vi "replace cursor - plot ref - V2.vi"(0 "Plot ref in":refnum<vi>, 1 "new X":dbl=nan, 3 "new  Y":dbl=nan, 5 "cursor index":i32, 6 "cursor action":T1=enum."write", 7 "label":enum16{"hide", "show x", "show y", "show (x,y)"}(ring), 9 "x-label":string, 11 "y-label":string, 12 "Color Box":u32(colorbox)=327424, 13 "cursor state":T2(ring)=enum."boring") -> (14 "Plot ref out":refnum<vi>, 15 "read X":dbl, 18 "read Y":dbl)   [LabVIEW 2015]
uses:
  cursor action.ctl
panel:
  in  "action":enum16{"", "read", "write"}(ring)=enum."write"
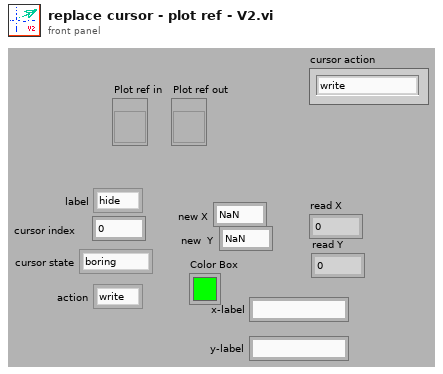
[diagram p1: front panel]
types:
  T1 = typedef "cursor action.ctl" = enum16{"range", "read", "write", "check", "zoom out", "smart zoom out"}
  T2 = enum16{"normal", "alert", "fuzzy", "interesting", "boring", "colored"}
  T3 = typedef "LVCursorListTypeDef.ctl" = cluster{"Name":string, "Color":u32, "Style":u8, "Point Style":u8, "Name Visible":bool, "Allow Drag":bool, "Cursor Mode":u32, "Plot":i32, "Index":i32, "Position":cluster{"X":dbl, "Y":dbl}, "X Scale":u32, "Y Scale":u32, "Watch Plots":i32[], "Watch All Plots":bool, "Plot Area":i32, "Label Offset":cluster{"X":dbl, "Y":dbl}}[]
  T4 = cluster{"Name":string, "Color":u32, "Style":u8, "Point Style":u8, "Name Visible":bool, "Allow Drag":bool, "Cursor Mode":u32, "Plot":i32, "Index":i32, "Position":cluster{"X":dbl, "Y":dbl}, "X Scale":u32, "Y Scale":u32, "Watch Plots":i32[], "Watch All Plots":bool, "Plot Area":i32, "Label Offset":cluster{"X":dbl, "Y":dbl}}
  T5 = typedef "LVRangeTypeDef.ctl" = cluster{"Minimum":dbl, "Maximum":dbl, "Increment":dbl, "Minor Increment":dbl, "Start":dbl}
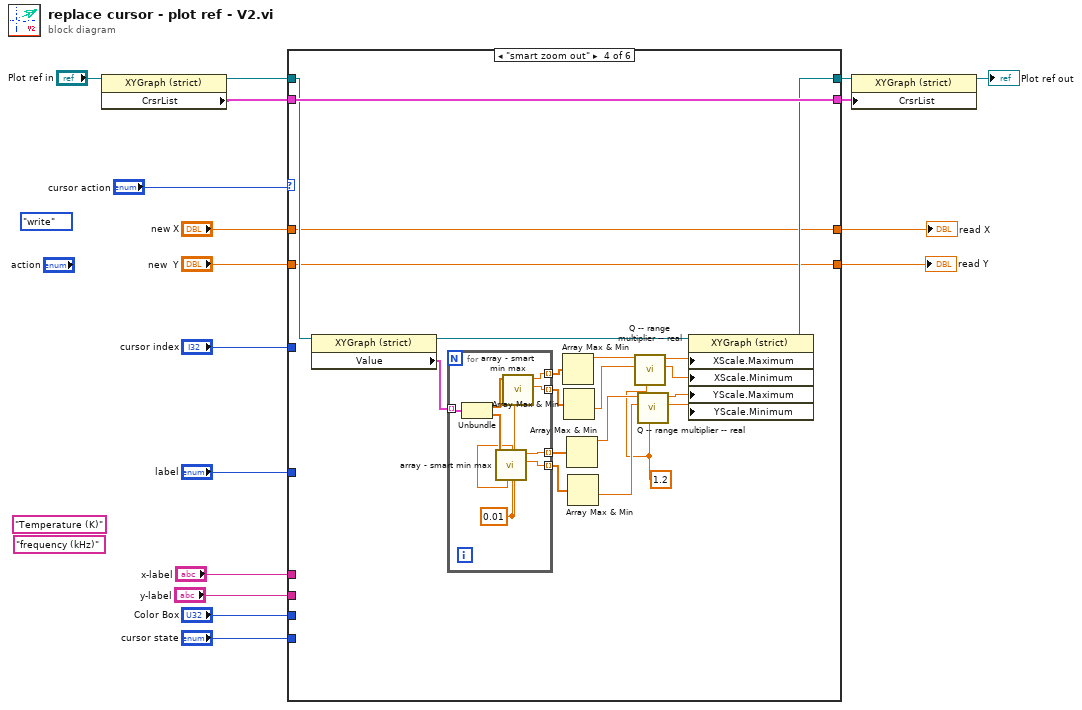
[diagram p0: block diagram]
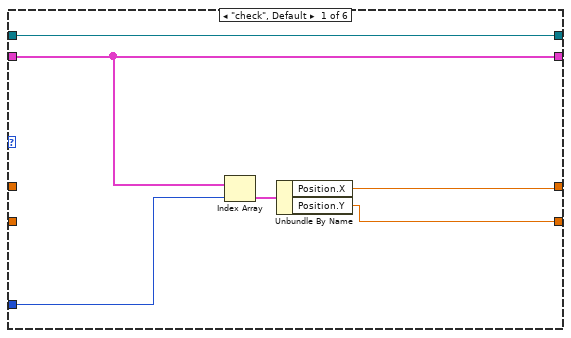
[diagram p2: hidden frame]
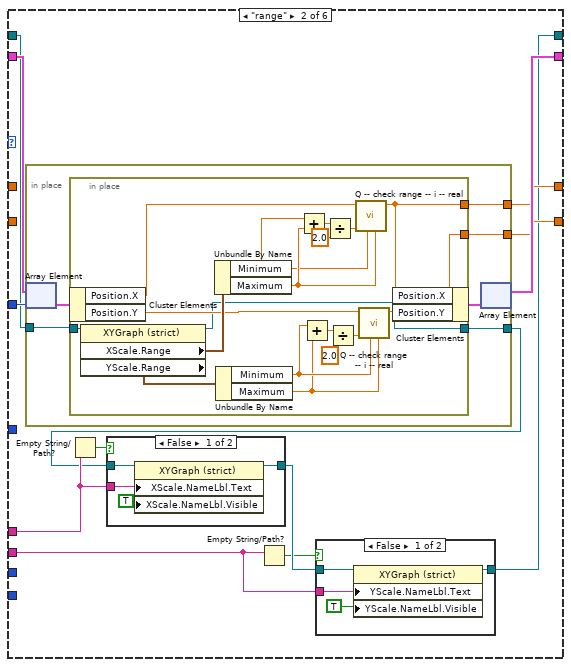
[diagram p3: hidden frame]
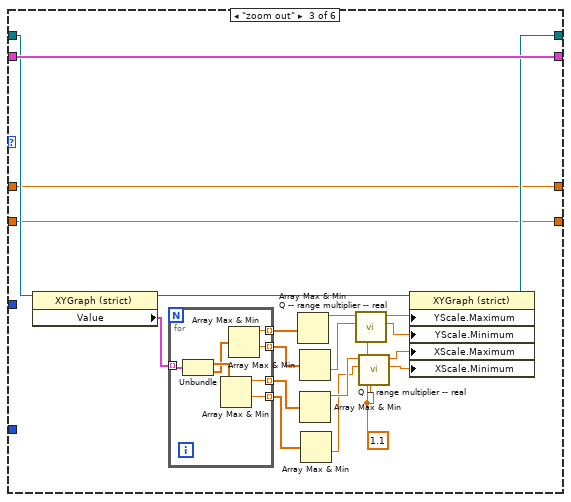
[diagram p6: hidden frame]
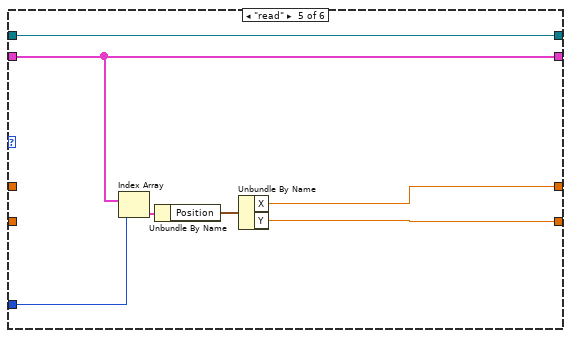
[diagram p7: hidden frame]
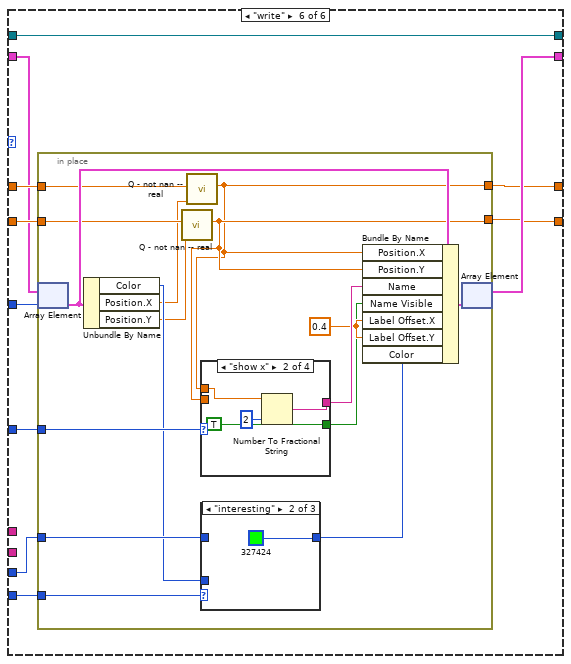
[diagram p8: hidden frame]
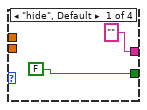
[diagram p11: hidden frame]
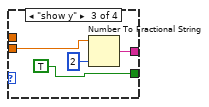
[diagram p12: hidden frame]
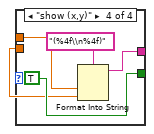
[diagram p13: hidden frame]
diagram:
  (unwired) "frequency (kHz)"
  (unwired) "Temperature (K)"
  (unwired) cursor_action."write" ("cursor action")
  n1 = property on="Property Node" class="XYGraph (strict)"(reference="Plot ref in") -> (reference out=w3:refnum<vi>, "CrsrList"=w12:T3)  [unwired: 1 in, 1 out]
  n2 = case shown="\"smart zoom out\"" "cursor action" {
    tunnel: "cursor index" -> [w21 w34 _ _ w131 w139]
    tunnel: w12 -> [w22 w36 w90 w117 w129 w141]
    tunnel: [w22 w35 w90 w117 w129 w140] -> w11
    tunnel: "new  Y" -> [_ _ w85 w112 _ w142]
    tunnel: "new X" -> [_ _ w86 w113 _ w143]
    tunnel: [w19 w33 w86 w113 w128 w138] -> w14
    tunnel: [w18 w32 w85 w112 w127 w137] -> w13
    tunnel: "label" -> [_ _ _ _ _ w136]
    tunnel: "Color Box" -> [_ _ _ _ _ w135]
    tunnel: "cursor state" -> [_ _ _ _ _ w134]
    tunnel: [w23 w24 w87 w114 w126 w133] -> w4
    tunnel: w3 -> [w23 w31 w89 w116 w126 w133]
    tunnel: "x-label" -> [_ w29 _ _ _ _]
    tunnel: "y-label" -> [_ w26 _ _ _ _]
    frame "check", Default {
      n3 = Index Array(array=w22, index=w21) -> (element=w20:T4)
      n4 = Unbundle By Name(w20) -> ("Position.X"=w19:dbl, "Position.Y"=w18:dbl)
    }
    frame "range" {
      n5 = in-place {
        in-place-border: w31 -> [w50]
        in-place-border: [w49] -> w33
        in-place-border: [w48] -> w32
        in-place-border: [w47] -> w25
        n6 = in-place-array #1(w36, w34) -> (w52:T4)
        n7 = in-place {
          in-place-border: w50 -> [w58]
          in-place-border: [w55] -> w49
          in-place-border: [w54] -> w48
          in-place-border: [w53] -> w47
          n8 = in-place-cluster #2(w52) -> ("Position.X"=w57:dbl, "Position.Y"=w56:dbl)
          n9 = property on="Property Node" class="XYGraph (strict)"(reference=w58) -> (reference out=w53:refnum<vi>, "XScale.Range"=w59:T5, "YScale.Range"=w60:T5)  [unwired: 1 in, 1 out]
          n10 = Unbundle By Name(w59) -> ("Minimum"=w61:dbl, "Maximum"=w62:dbl)
          n11 = Unbundle By Name(w60) -> ("Minimum"=w70:dbl, "Maximum"=w69:dbl)
          n12 = Add(x=w61, y=w62) -> (x+y=w63:dbl)
          n13 = Add(x=w70, y=w69) -> (x+y=w66:dbl)
          n14 = Divide(x=w63, y=2.0) -> (x/y=w65:dbl)
          n15 = Divide(x=w66, y=2.0) -> (x/y=w68:dbl)
          n16 = call "Q -- check range -- i -- real.vi"("upper"=w62, "lower"=w61, "default"=w65, "number"=w57) -> ("number in range"=w55:dbl)  [unwired: 5 in, 2 out]
          n17 = call "Q -- check range -- i -- real.vi"("upper"=w69, "lower"=w70, "default"=w68, "number"=w56) -> ("number in range"=w54:dbl)  [unwired: 5 in, 2 out]
          n18 = in-place-cluster #2("Position.X"=w55, "Position.Y"=w54) -> (w51:T4)
        }
        n19 = in-place-array #1(w51) -> (w35:T3)  [unwired: 1 out]
      }
      n20 = Empty String/Path?(string/path=w29) -> (empty?=w30:bool)
      n21 = case shown="False" w30 {
        tunnel: w25 -> [w45 w46]
        tunnel: w29 -> [w44 _]
        tunnel: [w43 w46] -> w28
        frame False {
          n22 = property on="Property Node" class="XYGraph (strict)"(reference=w45, "XScale.NameLbl.Text"=w44, "XScale.NameLbl.Visible"=TRUE ("X Scale.Name Label.Visible")) -> (reference out=w43:refnum<vi>)  [unwired: 1 in, 1 out]
        }
        frame True {
        }
      }
      n23 = Empty String/Path?(string/path=w26) -> (empty?=w27:bool)
      n24 = case shown="False" w27 {
        tunnel: w28 -> [w40 w41]
        tunnel: w26 -> [w39 _]
        tunnel: [w38 w41] -> w24
        frame False {
          n25 = property on="Property Node" class="XYGraph (strict)"(reference=w40, "YScale.NameLbl.Text"=w39, "YScale.NameLbl.Visible"=TRUE ("X Scale.Name Label.Visible")) -> (reference out=w38:refnum<vi>)  [unwired: 1 in, 1 out]
        }
        frame True {
        }
      }
    }
    frame "zoom out" {
      w71 = 1.1 ("factor")
      n26 = property on="Property Node" class="XYGraph (strict)"(reference=w89) -> (reference out=w88:refnum<vi>, "Value"=w84:cluster{dbl[], dbl[]}[])  [unwired: 1 in, 1 out]
      n27 = for {
        tunnel: w84 -> [w91] mode=indexing
        tunnel: [w92] -> w80 mode=indexing
        tunnel: [w93] -> w81 mode=indexing
        tunnel: [w94] -> w82 mode=indexing
        tunnel: [w95] -> w83 mode=indexing
        n28 = Unbundle(w91) -> (w97:dbl[], w96:dbl[])
        n29 = Array Max & Min(array=w97) -> (max value=w93:dbl, min value=w92:dbl)  [unwired: 2 out]
        n30 = Array Max & Min(array=w96) -> (max value=w95:dbl, min value=w94:dbl)  [unwired: 2 out]
      }
      n31 = Array Max & Min(array=w83) -> (max value=w75:dbl)  [unwired: 3 out]
      n32 = Array Max & Min(array=w82) -> (min value=w74:dbl)  [unwired: 3 out]
      n33 = Array Max & Min(array=w81) -> (max value=w73:dbl)  [unwired: 3 out]
      n34 = Array Max & Min(array=w80) -> (min value=w72:dbl)  [unwired: 3 out]
      n35 = call "Q -- range multiplier -- real.vi"("factor"=w71, "lower"=w74, "upper"=w75) -> ("lower OUT"=w76:dbl, "upper OUT"=w77:dbl)  [unwired: 5 in, 2 out]
      n36 = call "Q -- range multiplier -- real.vi"("factor"=w71, "lower"=w72, "upper"=w73) -> ("lower OUT"=w78:dbl, "upper OUT"=w79:dbl)  [unwired: 5 in, 2 out]
      n37 = property on="Property Node" class="XYGraph (strict)"(reference=w88, "YScale.Maximum"=w77, "YScale.Minimum"=w76, "XScale.Maximum"=w79, "XScale.Minimum"=w78) -> (reference out=w87:refnum<vi>)  [unwired: 1 in, 1 out]
    }
    frame "smart zoom out" {
      w98 = 1.2 ("factor")
      n38 = property on="Property Node" class="XYGraph (strict)"(reference=w116) -> (reference out=w115:refnum<vi>, "Value"=w111:cluster{dbl[], dbl[]}[])  [unwired: 1 in, 1 out]
      n39 = for {
        tunnel: w111 -> [w123] mode=indexing
        tunnel: [w122] -> w104 mode=indexing
        tunnel: [w124] -> w101 mode=indexing
        tunnel: [w119] -> w100 mode=indexing
        tunnel: [w125] -> w106 mode=indexing
        w118 = 0.01 ("median range")
        n40 = Unbundle(w123) -> (w121:dbl[], w120:dbl[])
        n41 = call "array - smart min max.vi"("median range"=w118, "x"=w120) -> ("min"=w122:dbl, "max"=w124:dbl)  [unwired: 8 in]
        n42 = call "array - smart min max.vi"("median range"=w118, "x"=w121) -> ("min"=w119:dbl, "max"=w125:dbl)  [unwired: 8 in]
      }
      n43 = Array Max & Min(array=w106) -> (max value=w105:dbl)  [unwired: 3 out]
      n44 = Array Max & Min(array=w100) -> (min value=w99:dbl)  [unwired: 3 out]
      n45 = Array Max & Min(array=w101) -> (max value=w102:dbl)  [unwired: 3 out]
      n46 = Array Max & Min(array=w104) -> (min value=w103:dbl)  [unwired: 3 out]
      n47 = call "Q -- range multiplier -- real.vi"("factor"=w98, "lower"=w99, "upper"=w105) -> ("lower OUT"=w107:dbl, "upper OUT"=w108:dbl)  [unwired: 5 in, 2 out]
      n48 = call "Q -- range multiplier -- real.vi"("factor"=w98, "lower"=w103, "upper"=w102) -> ("lower OUT"=w109:dbl, "upper OUT"=w110:dbl)  [unwired: 5 in, 2 out]
      n49 = property on="Property Node" class="XYGraph (strict)"(reference=w115, "XScale.Maximum"=w108, "XScale.Minimum"=w107, "YScale.Maximum"=w110, "YScale.Minimum"=w109) -> (reference out=w114:refnum<vi>)  [unwired: 1 in, 1 out]
    }
    frame "read" {
      n50 = Index Array(array=w129, index=w131) -> (element=w132:T4)
      n51 = Unbundle By Name(w132) -> ("Position"=w130:cluster{"X":dbl, "Y":dbl})
      n52 = Unbundle By Name(w130) -> ("X"=w128:dbl, "Y"=w127:dbl)
    }
    frame "write" {
      n53 = in-place {
        in-place-border: w143 -> [w146]
        in-place-border: w142 -> [w149]
        in-place-border: [w145] -> w138
        in-place-border: [w147] -> w137
        in-place-border: w136 -> [w155]
        in-place-border: w135 -> [w152]
        in-place-border: w134 -> [w153]
        w156 = 0.4 ("Label Offset.X")
        n54 = in-place-array #3(w141, w139) -> (w159:T4)
        n55 = Unbundle By Name(w159) -> ("Color"=w150:u32, "Position.X"=w144:dbl, "Position.Y"=w148:dbl)
        n56 = call "Q - not nan -- real.vi"("default"=w148, "Numeric"=w149) -> ("out"=w147:dbl)  [unwired: 8 in, 1 out]
        n57 = call "Q - not nan -- real.vi"("default"=w144, "Numeric"=w146) -> ("out"=w145:dbl)  [unwired: 8 in, 1 out]
        n58 = case shown="\"show x\"" w155 {
          tunnel: w145 -> [_ w168 _ w174]
          tunnel: ["" ("format string") w167 w171 w177] -> w158
          tunnel: [FALSE ("Name Visible") TRUE ("Name Visible") TRUE ("Name Visible") TRUE ("Name Visible")] -> w154
          tunnel: w147 -> [_ _ w170 w173]
          frame "hide", Default {
          }
          frame "show x" {
            n59 = Number To Fractional String(number=w168, precision (6)=i16 2) -> (F-format string=w167:string)  [unwired: 2 in]
          }
          frame "show y" {
            n60 = Number To Fractional String(number=w170, precision (6)=i16 2) -> (F-format string=w171:string)  [unwired: 2 in]
          }
          frame "show (x,y)" {
            n61 = Format Into String(format string="(%4f\\n%4f)", w174, w173) -> (resulting string=w177:string)  [unwired: 2 in, 1 out]
          }
        }
        n62 = case shown="\"interesting\"" w153 {
          tunnel: [w160 u32 327424 ("Color Box") w162] -> w151
          tunnel: w152 -> [_ _ w162]
          tunnel: w150 -> [w160 _ _]
          frame "boring", Default {
          }
          frame "interesting" {
          }
          frame "colored" {
          }
        }
        n63 = Bundle By Name(cluster=w159, "Position.X"=w145, "Position.Y"=w147, "Name"=w158, "Name Visible"=w154, "Label Offset.X"=w156, "Label Offset.Y"=w156, "Color"=w151) -> (w157:T4)
        n64 = in-place-array #3(w157) -> (w140:T3)  [unwired: 1 out]
      }
    }
  }
  "read X" <- w14
  "read Y" <- w13
  n65 = property on="Property Node" class="XYGraph (strict)"(reference=w4, "CrsrList"=w11) -> (reference out=→"Plot ref out":refnum<vi>)  [unwired: 1 in, 1 out]
